vi "储运信息簇.vi"(0 "纬度":dbl, 1 "经度":dbl, 2 "温度":dbl, 3 "编号":i32, 4 "时间":timestamp) -> (5 "待写入的簇":T1 {"记录时间" format="%<%H:%M:%S\n%Y/%m/%d>T"})   [LabVIEW 2018]
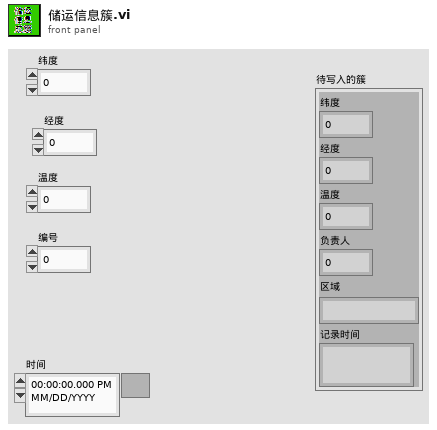
[diagram p1: front panel]
types:
  T1 = typedef "储运信息.ctl" = cluster{"纬度":sgl, "经度":sgl, "温度":sgl, "负责人":i32, "区域":string, "记录时间":timestamp}
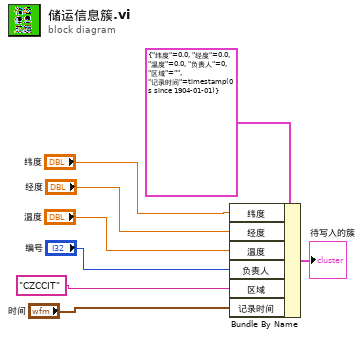
[diagram p0: block diagram]
diagram:
  n1 = Bundle By Name(cluster=T1 {"纬度"=0.0, "经度"=0.0, "温度"=0.0, "负责人"=0, "区域"="", "记录时间"=timestamp(0 s since 1904-01-01)} ("簇"), "纬度"="纬度", "经度"="经度", "温度"="温度", "负责人"="编号", "区域"="CZCCIT", "记录时间"="时间") -> (→"待写入的簇":T1)
